vi "Publish Current Build.vi"(8 "error in (no error)":errorcluster, 9 "Build Specification Name":string, 10 "Target":string, 11 "CD Build Tools in":refnum<class "Project Build Tools.lvclass">) -> (0 "error out":errorcluster, 3 "CD Build Tools out":refnum<class "Project Build Tools.lvclass">)   [LabVIEW 2019, in "Project Build Tools.lvclass"]
uses:
  Project Build Tools.lvclass
  Project Build Tools.lvclass/Project Build Tools.ctl
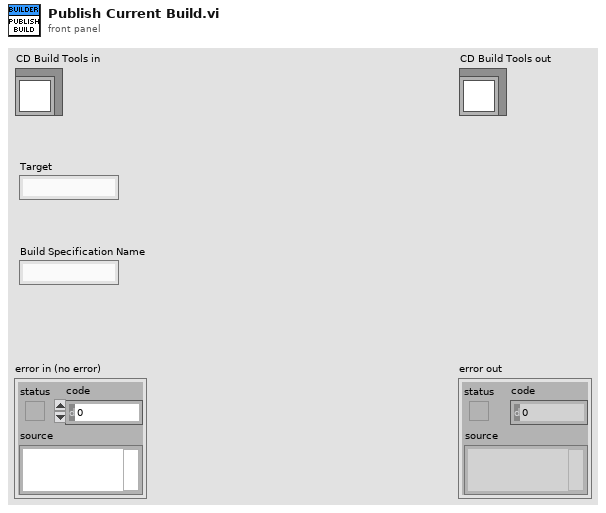
[diagram p1: front panel]
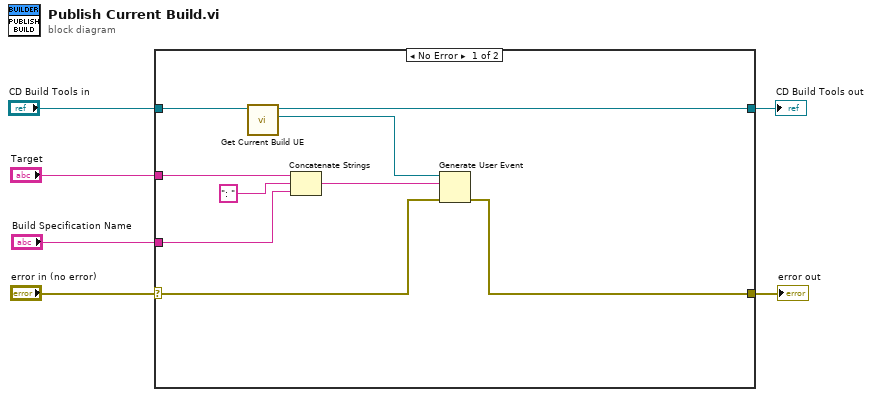
[diagram p0: block diagram]
diagram:
  n1 = case shown="No Error" "error in (no error)" {
    selector: "error in (no error)" -> [w8 w17]
    tunnel: [w7 w17] -> w5
    tunnel: [w14 w16] -> w3
    tunnel: "CD Build Tools in" -> [w15 w16]
    tunnel: "Target" -> [w11 _]
    tunnel: "Build Specification Name" -> [w10 _]
    frame No Error {
      n2 = call "Get Current Build UE.vi"("CD Build Tools in"=w15) -> ("Current Build UE"=w13:refnum<user-event>, "CD Build Tools out"=w14:refnum<class "Project Build Tools.lvclass">)  [unwired: 9 in]
      n3 = Concatenate Strings(w11, ": " ("string"), w10) -> (w9:string)
      n4 = Generate User Event(user event=w13, event data cluster=w9, error in=w8) -> (error out=w7:errorcluster)  [unwired: 1 in, 1 out]
    }
    frame Error {
    }
  }
  "error out" <- w5
  "CD Build Tools out" <- w3
